vi "Load Config.vi"(6 "Constants":refnum<class "Sequence Constants.lvclass">, 8 "error in (no error)":refnum<class "MultiErrors.lvclass">, 10 "Config Element":refnum<class "Config Element.lvclass">, 11 "Stop Seq Command Config in":refnum<class "Stop Seq Command Config.lvclass">) -> (0 "error out":refnum<class "MultiErrors.lvclass">, 3 "Stop Seq Command Config out":refnum<class "Stop Seq Command Config.lvclass">)   [LabVIEW 2020, in "VolatusSeqConfig.lvlib" / "Stop Seq Command Config.lvclass"]
uses:
  Stop Seq Command Config.lvclass
  VolatusErrorUtilities/MultiErrors/MultiErrors.lvclass
  lv-cdm/CDM-Config/Config Element/Config Element.lvclass
  Stop Seq Command Config.lvclass/Stop Seq Command Config.ctl
  Sequence Constants/Sequence Constants.lvclass
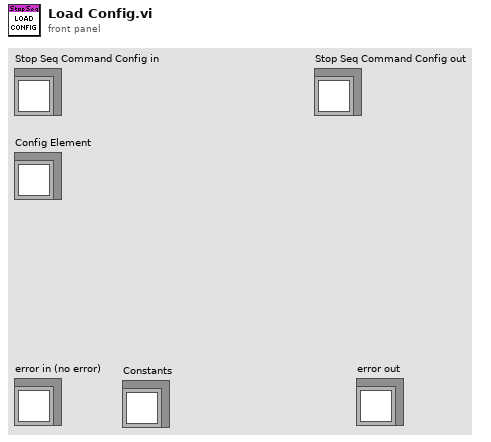
[diagram p1: front panel]
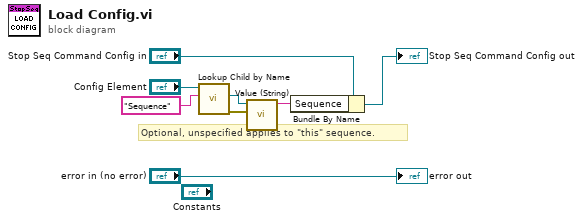
[diagram p0: block diagram]
diagram:
  # "Optional, unspecified applies to \"this\" sequence."
  n1 = call "Lookup Child by Name.vi"("Name"="Sequence", "Config Element in"="Config Element") -> ("error out"=w4:errorcluster, "Child"=w3:refnum<class "Config Element.lvclass">)  [unwired: 6 in, 2 out]
  n2 = call "Value (String).vi"("error in (no error)"=w4, "Config Element in"=w3) -> ("String Value"=w1:string)  [unwired: 8 in, 1 out]
  n3 = Bundle By Name(cluster="Stop Seq Command Config in", "Sequence"=w1) -> (→"Stop Seq Command Config out":refnum<class "Stop Seq Command Config.lvclass">)
  "error out" <- "error in (no error)"
